vi "LV8_4.vi"() -> ()   [LabVIEW 2016]
uses:
  <vilib>/imath/engines/lvmath2/RunTimeEngine/BuiltInFunctions/randnormal/NIMS_randnormal(Str,I32).vi
  <vilib>/imathl/engines/lvmath/Functions/Error Handling/Create Error.vi
  <vilib>/imath/engines/lvmath2/RunTimeEngine/BuiltInFunctions/randnormal/NIMS_randnormal(1,I32).vi
  <vilib>/imath/engines/lvmath2/RunTimeEngine/ErrorHandling/NIMS_Error From Error Code.vi
  <vilib>/imath/engines/lvmath2/RunTimeEngine/RangeToken/NIMS_Range_R2 - Integer.vi
  <instcachedir>/0/NIMS_Range_R2 - Integer_89B873E74E6E489885E44F751DD9C6BF.lvgen/NIMS_Range_R2 - Integer_89B873E74E6E489885E44F751DD9C6BF_000.vi
  <vilib>/imath/engines/lvmath2/RunTimeEngine/CommandStatement/MC_CommandStatement_break.vi
  <vilib>/imath/engines/lvmath2/RunTimeEngine/IndexRead/NIMS V(S).vi
  <instcachedir>/0/NIMS V(S)_0488751826AF41519A22953C041130DC.lvgen/NIMS V(S)_0488751826AF41519A22953C041130DC_000.vi
  <vilib>/imath/engines/lvmath2/RunTimeEngine/RangeToken/NIMS_Range.vi
  <instcachedir>/0/NIMS_Range_A7C094595B484CA7AF10685B02D808ED.lvgen/NIMS_Range_A7C094595B484CA7AF10685B02D808ED_001.vi
  <vilib>/imath/engines/lvmath2/RunTimeEngine/BuiltInFunctions/poly/NIMS_GV=poly(GV).vi
  <instcachedir>/0/NIMS_GV=poly(GV)_A1C8B7C92C4F409DB664B03EC1C81090.lvgen/NIMS_GV=poly(GV)_A1C8B7C92C4F409DB664B03EC1C81090_000.vi
  <vilib>/imath/engines/lvmath2/RunTimeEngine/BuiltInFunctions/filter/NIMS_filter(GV,GV,GV,GV,Str).vi
  <instcachedir>/0/NIMS_filter(GV,GV,GV,GV,Str)_434E59EE96884CB3BC5141C85D3A0B2F.lvgen/NIMS_filter(GV,GV,GV,GV,Str)_434E59EE96884CB3BC5141C85D3A0B2F_002.vi
  <vilib>/imath/engines/lvmath2/RunTimeEngine/BuiltInFunctions/linramp/NIMS_linramp.vi
  <vilib>/imath/engines/lvmath2/RunTimeEngine/BuiltInFunctions/polyval/NIMS_polyval(GV,GM).vi
  <instcachedir>/0/NIMS_polyval(GV,GM)_E12556DC54744E0C81968744501C4F35.lvgen/NIMS_polyval(GV,GM)_E12556DC54744E0C81968744501C4F35_003.vi
  <vilib>/imath/engines/lvmath2/RunTimeEngine/ArithmeticOperatorToken/NIMS_ArithmeticOperator_rightdiv(C,C).vi
  <instcachedir>/0/NIMS_ArithmeticOperator_rightdiv(C,C)_6F3C2C239EC94040B0793F3E73F9E5CA.lvgen/NIMS_ArithmeticOperator_rightdiv(C,C)_6F3C2C239EC94040B0793F3E73F9E5CA_000.vi
  <vilib>/imath/engines/lvmath2/RunTimeEngine/BuiltInFunctions/fft/NIMS_fft(GV).vi
  <instcachedir>/0/NIMS_fft(GV)_4C6467FC22F84E4BA42517A07EF978B0.lvgen/NIMS_fft(GV)_4C6467FC22F84E4BA42517A07EF978B0_000.vi
  <vilib>/imath/engines/lvmath2/RunTimeEngine/BuiltInFunctions/fftshift/NIMS_fftshift(GV).vi
  <instcachedir>/0/NIMS_fftshift(GV)_BD7A7BA9CA6B470B9A9F73A6A3FEEB3E.lvgen/NIMS_fftshift(GV)_BD7A7BA9CA6B470B9A9F73A6A3FEEB3E_000.vi
  <vilib>/imath/engines/lvmath2/RunTimeEngine/BuiltInFunctions/abs/NIMS_abs(signed).vi
  <instcachedir>/0/NIMS_abs(signed)_C4FCB8E6058B49B797C7C8D53CA5F6EC.lvgen/NIMS_abs(signed)_C4FCB8E6058B49B797C7C8D53CA5F6EC_006.vi
  <instcachedir>/0/NIMS_fft(GV)_4C6467FC22F84E4BA42517A07EF978B0.lvgen/NIMS_fft(GV)_4C6467FC22F84E4BA42517A07EF978B0_001.vi
  <vilib>/imath/engines/lvmath2/RunTimeEngine/IndexRead/NIMS V(R2).vi
  <instcachedir>/0/NIMS V(R2)_C76619605A0E4E9F8B2FA9389712AC47.lvgen/NIMS V(R2)_C76619605A0E4E9F8B2FA9389712AC47_000.vi
  <vilib>/imath/engines/lvmath2/RunTimeEngine/NodeEndStatement/NIMS_NodeEndStatement_Output.vi
  <instcachedir>/0/NIMS_NodeEndStatement_Output_53EC0D466D134D7ABD903AC30B43404B.lvgen/NIMS_NodeEndStatement_Output_53EC0D466D134D7ABD903AC30B43404B_000.vi
  <instcachedir>/0/NIMS_NodeEndStatement_Output_53EC0D466D134D7ABD903AC30B43404B.lvgen/NIMS_NodeEndStatement_Output_53EC0D466D134D7ABD903AC30B43404B_005.vi
  <instcachedir>/0/NIMS_NodeEndStatement_Output_53EC0D466D134D7ABD903AC30B43404B.lvgen/NIMS_NodeEndStatement_Output_53EC0D466D134D7ABD903AC30B43404B_004.vi
  <vilib>/imath/engines/lvmath2/RunTimeEngine/ErrorHandling/NIMS_Finalize Error.vi
panel:
  out "Pole-Zero Plot":cluster{dbl[], dbl[]}[](graph)=[{array[401 elements], array[401 elements]}, {[1.0, 0.7071067811865477, 0.7071067811865477, -3.51308055362512e-16, -3.51308055362512e-16], [0.0, 0.7071067811865472, -0.7071067811865472, -1.0, 1.0]}, {[0.9499999999999996, -2.1378419577758464e-16, -2.1378419577758464e-16, 0.6717514421272202, 0.6717514421272202], [0.0, -0.95, 0.95, 0.6717514421272204, -0.6717514421272204]}]
  in  "# of interference harmonics":i32(slide)=2 scale=1.0..3.0
  in  "pole radius":dbl(slide)=0.95 scale=0.5..0.99
  in  "interference frequency":dbl(slide)=60.0 scale=40.0..80.0
  out "Filtered (freq domain)":cluster{"F":dbl[], "FYI":dbl[]}(graph)
  out "Original signal (freq domain)":cluster{"F":dbl[], "H":dbl[]}[](graph)
  out "Original signal (time domain)":cluster{"N":i32[], "X":dbl[]}(graph)={"N"=[1, 2, 3, 4, 5, 6, 7, 8, 9, 10, 11, 12, 13, 14, 15, 16, 17, 18, 19, 20, 21, 22, 23, 24, 25, 26, 27, 28, 29, 30, 31, 32, 33, 34, 35, 36, 37, 38, 39, 40, 41, 42, 43, 44, 45, 46, 47, 48, 49, 50, 51, 52, 53, 54, 55, 56, 57, 58, 59, 60, 61, 62, 63, 64, 65, 66, 67, 68, 69, 70, 71, 72, 73, 74, 75, 76, 77, 78, 79, 80, 81, 82, 83, 84, 85, 86, 87, 88, 89, 90, 91, 92, 93, 94, 95, 96, 97, 98, 99, 100], "X"=[1.7512456999983255, 0.18405864128361016, -0.4446827351219487, -0.6470243152058823, -1.2100495998521283, -1.2301549210894844, -0.09651336502424834, 0.6931205950117569, -0.09651336502424931, -1.2301549210894855, -1.2100495998521288, -0.6470243152058837, -0.4446827351219495, 0.18405864128360905, 1.751245699998326, 2.6931205950117567, 1.751245699998325, 0.18405864128360905, -0.44468273512194817, -0.6470243152058823, -1.2100495998521268, -1.2301549210894827, -0.09651336502424407, 0.6931205950117569, -0.09651336502424825, -1.2301549210894867, -1.2100495998521288, -0.6470243152058848, -0.4446827351219506, 0.18405864128361038, 1.7512456999983281, 2.6931205950117567, 1.7512456999983264, 0.1840586412836105, -0.4446827351219477, -0.6470243152058821, -1.2100495998521266, -1.230154921089483, -0.09651336502424425, 0.6931205950117569, -0.0965133650242549, -1.2301549210894875, -1.21004959985213, -0.647024315205885, -0.4446827351219523, 0.1840586412836137, 1.7512456999983266, 2.6931205950117567, 1.751245699998334, 0.18405864128360994, -0.4446827351219467, -0.6470243152058799, -1.2100495998521263, -1.230154921089479, -0.0965133650242451, 0.6931205950117569, -0.09651336502425405, -1.230154921089487, -1.2100495998521303, -0.6470243152058852, -0.44468273512195067, 0.18405864128361304, 1.7512456999983255, 2.6931205950117567, 1.7512456999983215, 0.18405864128361327, -0.44468273512194495, -0.6470243152058797, -1.210049599852126, -1.2301549210894795, -0.09651336502424594, 0.6931205950117569, -0.0965133650242532, -1.2301549210894869, -1.2100495998521326, -0.6470243152058854, -0.4446827351219525, 0.18405864128360983, 1.751245699998338, 2.6931205950117567, 1.7512456999983228, 0.18405864128360572, -0.4446827351219433, -0.6470243152058759, -1.2100495998521272, -1.2301549210894884, -0.09651336502426011, 0.6931205950117569, -0.09651336502425091, -1.2301549210894889, -1.2100495998521308, -0.6470243152058857, -0.4446827351219542, 0.18405864128360905, 1.751245699998349, 2.6931205950117567, 1.7512456999983104, 0.18405864128362304, -0.44468273512194306, -0.6470243152058828]}
  out "Filtered signal (time domain)":cluster{"N":i32[], "Y":dbl[]}(graph)={"N"=[1, 2, 3, 4, 5, 6, 7, 8, 9, 10, 11, 12, 13, 14, 15, 16, 17, 18, 19, 20, 21, 22, 23, 24, 25, 26, 27, 28, 29, 30, 31, 32, 33, 34, 35, 36, 37, 38, 39, 40, 41, 42, 43, 44, 45, 46, 47, 48, 49, 50, 51, 52, 53, 54, 55, 56, 57, 58, 59, 60, 61, 62, 63, 64, 65, 66, 67, 68, 69, 70, 71, 72, 73, 74, 75, 76, 77, 78, 79, 80, 81, 82, 83, 84, 85, 86, 87, 88, 89, 90, 91, 92, 93, 94, 95, 96, 97, 98, 99, 100], "Y"=[1.751245699998325, -0.027335414715562223, -0.3687685907250102, -0.5593651332804107, -1.2370330952850663, -1.0907639973677785, 0.07005511295888756, 0.4552472989273946, -0.5386910858650495, -1.306488221541407, -0.9247119334751979, -0.33933406592151094, -0.08192453085979046, 0.6096339216900941, 1.7712874553148186, 2.1557873306183972, 1.3431245909348917, 0.42160236951227237, 0.06659052624630535, -0.25688134441215765, -0.7930989063292303, -0.9288254440023301, -0.5497031745197705, -0.42357361057445564, -0.8094469680580836, -1.0086537231070267, -0.6358858003284669, -0.13866014025258666, 0.21259048024124827, 0.7170672666061255, 1.3601271449407522, 1.5727595838108324, 1.1634996067963388, 0.6191918609163714, 0.25820368406606553, -0.12375016209640155, -0.5977116306434678, -0.8575519679833081, -0.8224753249570784, -0.8103661298150198, -0.9286138525055805, -0.8775688175015324, -0.5087657165270216, -0.050338193862645486, 0.3422143909450891, 0.7643515468061394, 1.1791645272539861, 1.316153523876876, 1.0844418609208206, 0.7061562655286537, 0.3425377448871203, -0.0651555783300991, -0.5117164798989522, -0.8261826104198242, -0.9425296228300362, -0.980603832767799, -0.9810623763710662, -0.8198748546868555, -0.4528167775247618, -0.011465349829204552, 0.3992653309407841, 0.7851626195301626, 1.0995180531810065, 1.2032143535622888, 1.0496464385974964, 0.7444316192219511, 0.37965541413017134, -0.039366539375999876, -0.47386772068156524, -0.812376119577667, -0.9953687210101849, -1.0555299858473275, -1.0041463704556794, -0.7944822030319116, -0.42819215738709726, 0.005643625516257078, 0.42437497110454087, 0.7943221276392544, 1.0644635158774198, 1.1535068127714343, 1.0343320452860083, 0.7612776231344376, 0.395991890242233, -0.02801609557339446, -0.45720947237460696, -0.8062995147575405, -1.0186246172667945, -1.0885069839971182, -1.0143062518713184, -0.7833062198507883, -0.4173542053590882, 0.013173741839097586, 0.4354263933808602, 0.7983534714298007, 1.049035079152866, 1.1316291984362787, 1.027591772375387, 0.7686919987165619, 0.40318200905094437, -0.023020462554841137]}
  in  "stop":bool
  # "f = 30 Hz"
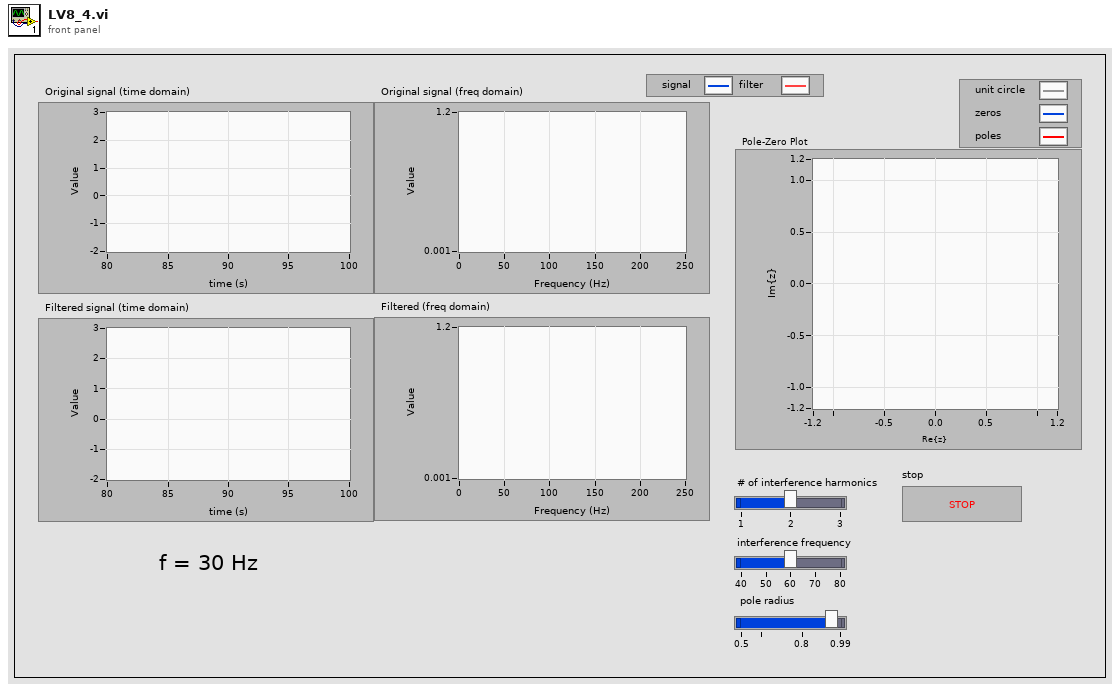
[diagram p1: front panel]
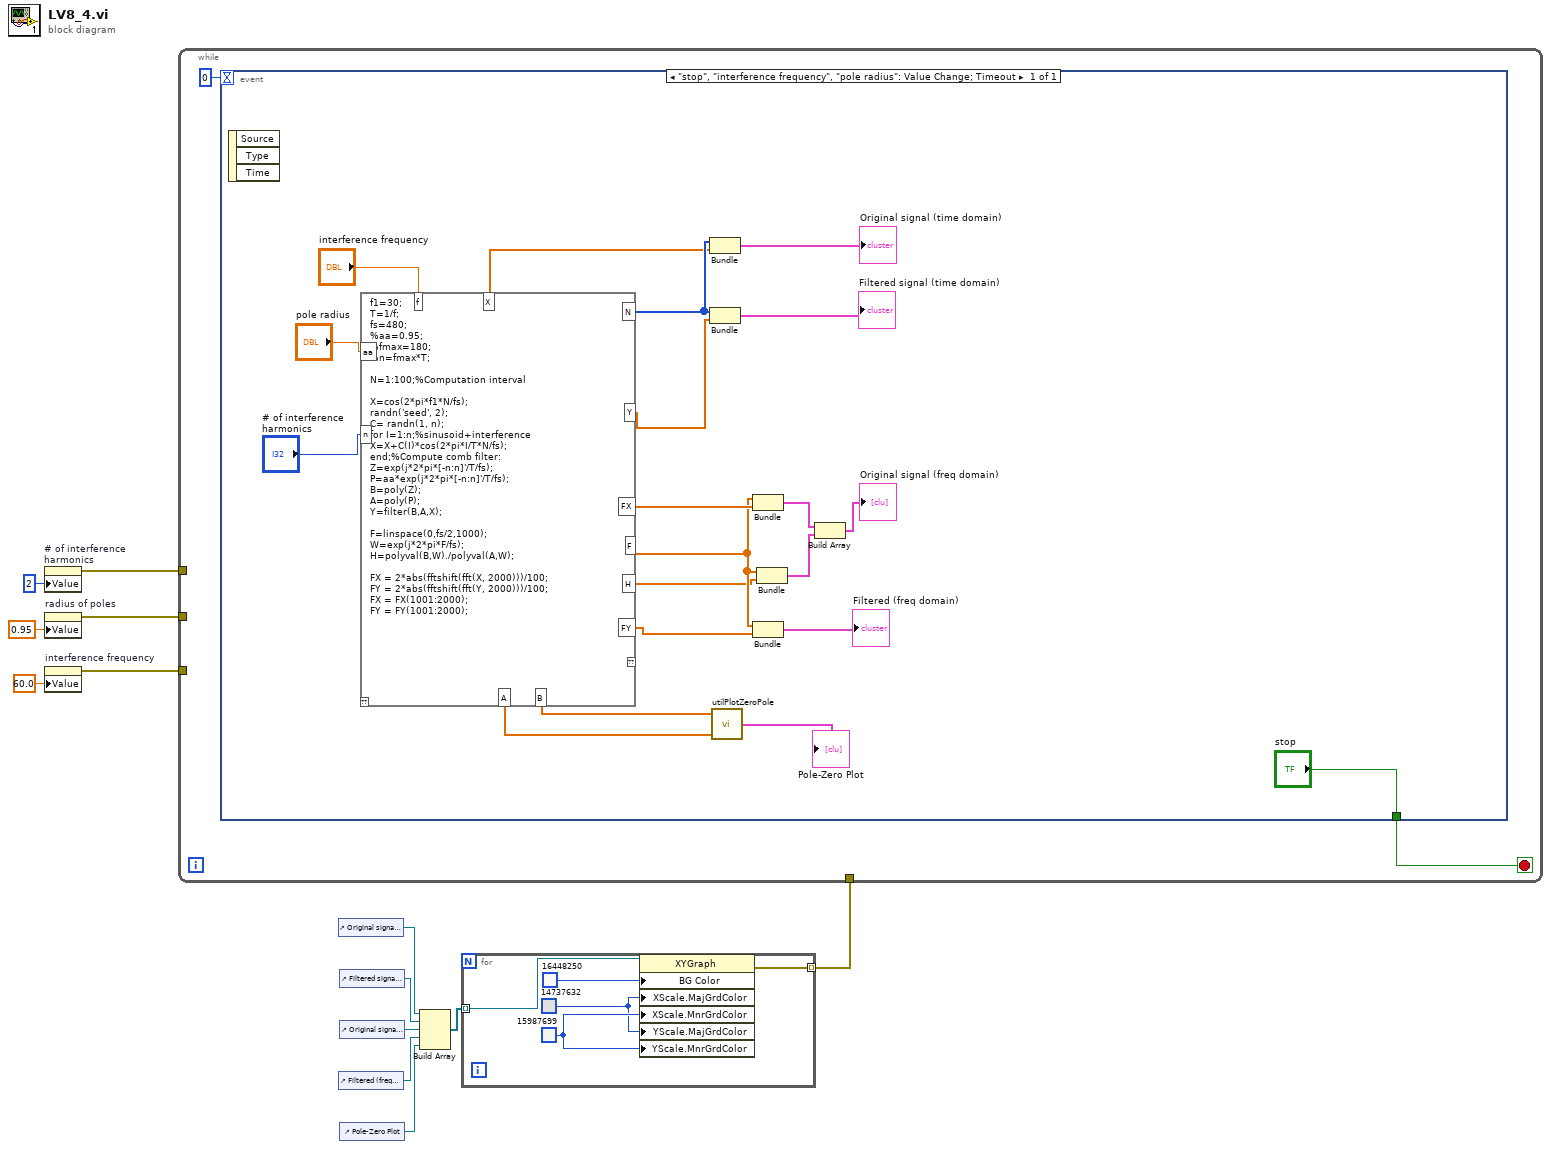
[diagram p0: block diagram]
diagram:
  n1 = property on="# of interference harmonics" class="Slide (strict)"("Value"=2 ("order")) -> (error out=w13:errorcluster)  [unwired: 2 in, 1 out]
  n2 = property on="radius of poles" class="Slide (strict)"("Value"=0.95 ("minus real part of poles")) -> (error out=w12:errorcluster)  [unwired: 2 in, 1 out]
  n3 = property on="interference frequency" class="Slide (strict)"("Value"=60.0 ("fundamental frequency")) -> (error out=w11:errorcluster)  [unwired: 2 in, 1 out]
  n4 = control-ref of="Original signal (time domain)"() -> (w6:refnum<vi>)
  n5 = control-ref of="Filtered (freq domain)"() -> (w3:refnum<vi>)
  n6 = control-ref of="Filtered signal (time domain)"() -> (w5:refnum<vi>)
  n7 = control-ref of="Original signal (freq domain)"() -> (w4:refnum<vi>)
  n8 = control-ref of="Pole-Zero Plot"() -> (w2:refnum<vi>)
  n9 = Build Array(w6, w5, w4, w3, w2) -> (w7:refnum<vi>[])
  n10 = for {
    tunnel: w7 -> [w15] mode=indexing
    tunnel: [w14] -> w1 mode=indexing
    w17 = u32 15987699
    w16 = u32 14737632
    n11 = property class="XYGraph"(reference=w15, "BG Color"=u32 16448250, "XScale.MajGrdColor"=w16, "XScale.MnrGrdColor"=w17, "YScale.MajGrdColor"=w16, "YScale.MnrGrdColor"=w17) -> (error out=w14:errorcluster)  [unwired: 1 in, 1 out]
  }
  n12 = while {
    tunnel: w13 -> [_]
    tunnel: w12 -> [_]
    tunnel: w11 -> [_]
    tunnel: w1 -> [_]
    stop <- w20 stop-if-true
    n13 = event shown="[0] \"stop\", \"interference frequency\", \"pole radius\": Value Change;  Timeout" {
      selector: _ -> [_]
      dyn-events: _ -> [_]
      timeout: 0 -> [_]
      tunnel: ["stop"] -> w20
      event "stop", "interference frequency", "pole radius": Value Change; Timeout {
        n14 = event-data() -> ()  [unwired: 1 in, 3 out]
        n15 = mathscript code="f1=30;\nT=1/f;\nfs=480;\n%aa=0.95;\n%fmax=180;\n%n=fmax*T;\n\nN=1:100;%Computation interval\n\nX=cos(2*pi*f1*N/fs);\nrandn('seed', 2);\nC= randn(1, n);\nfor I=1:n;%sinusoid+interference\nX=X+C(I)*cos(2*pi*I/T*N/fs);\nend;%Compute comb filter:\nZ=exp(j*2*pi*[-n:n]'/T/fs);\nP=aa*exp(j*2*pi*[-n:n]'/T/fs);\nB=poly(Z);\nA=poly(P);\nY=filter(B,A,X);\n\nF=linspace(0,fs/2,1000);\nW=exp(j*2*pi*F/fs);\nH=polyval(B,W)./polyval(A,W);\n\nFX = 2*abs(fftshift(fft(X, 2000)))/100;\nFY = 2*abs(fftshift(fft(Y, 2000)))/100;\nFX = FX(1001:2000);\nFY = FY(1001:2000);"("aa"="pole radius", "f"="interference frequency", "n"="# of interference harmonics") -> ("Y"=w30:cdb[], "F"=w37:dbl[], "FY"=w29:dbl[], "N"=w34:i32[], "FX"=w38:dbl[], "H"=w27:cdb[], "X"=w31:dbl[], "B"=w22:cdb[], "A"=w21:cdb[])  [unwired: 1 in, 1 out]
        n16 = Bundle("N"=w34, "X"=w31) -> (→"Original signal (time domain)":cluster{"N":i32[], "X":dbl[]})  [unwired: 1 in]
        n17 = Bundle("N"=w34, "Y"=w30) -> (→"Filtered signal (time domain)":cluster{"N":i32[], "Y":cdb[]})  [unwired: 1 in]
        n18 = call "utilPlotZeroPole.vi"("a, reverse coefficients"=w21, "b, forward coefficients"=w22) -> ("Pole-Zero Plot"=→"Pole-Zero Plot":cluster{dbl[], dbl[]}[])  [unwired: 3 in]
        n19 = Bundle("F"=w37, "FX"=w38) -> (w26:cluster{"F":dbl[], "FX":dbl[]})  [unwired: 1 in]
        n20 = Bundle("F"=w37, "FY"=w29) -> (→"Filtered (freq domain)":cluster{"F":dbl[], "FY":dbl[]})  [unwired: 1 in]
        n21 = Bundle("F"=w37, "H"=w27) -> (w25:cluster{"F":dbl[], "H":cdb[]})  [unwired: 1 in]
        n22 = Build Array(w26, w25) -> (→"Original signal (freq domain)":cluster{"F":dbl[], "H":cdb[]}[])
      }
    }
  }
